vi "load_config.vi"(8 "error in (no error)":errorcluster, 11 "Path":path) -> (0 "error out":errorcluster, 3 "Config Settings":T1)   [LabVIEW 2024]
uses:
  controls/Config_Settings.ctl
  <vilib>/Utility/config.llb/Read Key (Double).vi
  <vilib>/Utility/config.llb/Read Key (U32).vi
  <vilib>/Utility/config.llb/NI_LVConfig.lvlib
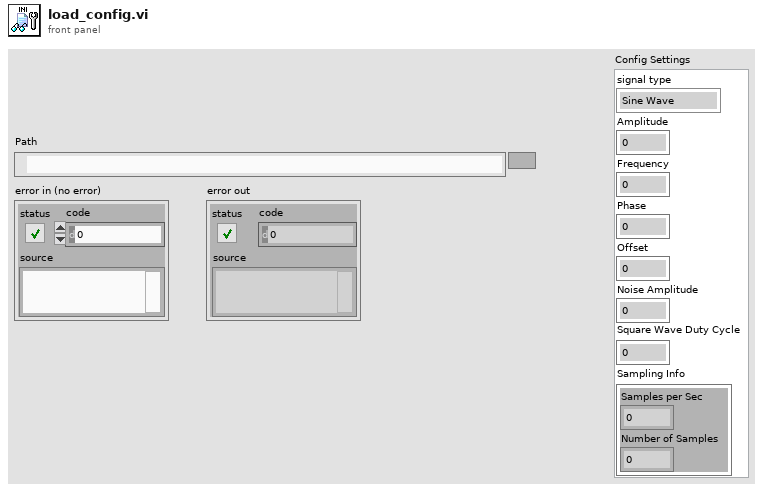
[diagram p1: front panel]
types:
  T1 = typedef "Config_Settings.ctl" = cluster{"signal type":enum16{"Sine Wave", "Triangle Wave", "Square Wave", "Sawtooth Wave"}, "Amplitude":dbl, "Frequency":dbl, "Phase":dbl, "Offset":dbl, "Noise Amplitude":dbl, "Square Wave Duty Cycle":dbl, "Sampling Info":cluster{"Samples per Sec":dbl, "Number of Samples":dbl}}
  T2 = enum16{"Sine Wave", "Triangle Wave", "Square Wave", "Sawtooth Wave"}
  T3 = typedef "NI_LVConfig.lvlib/Config Data RefNum.ctl" = refnum<k1>
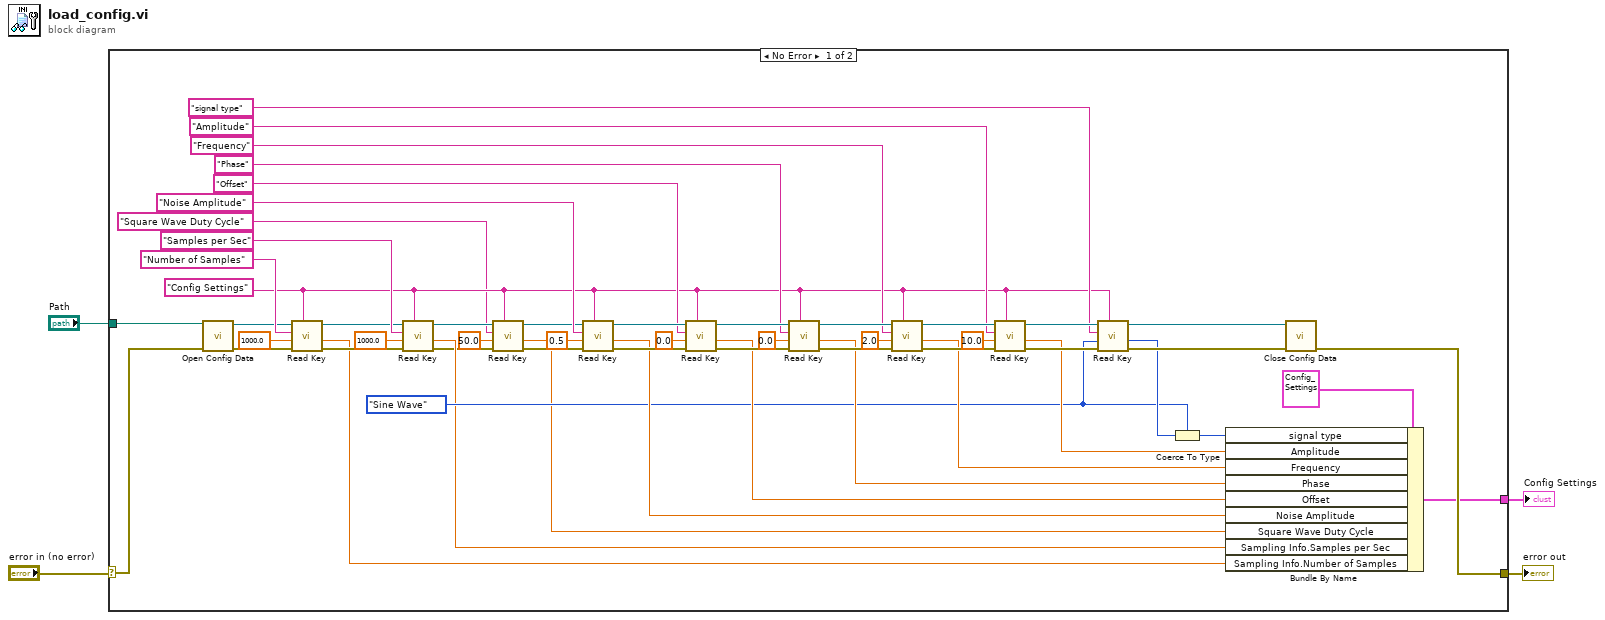
[diagram p0: block diagram]
diagram:
  n1 = case shown="No Error" "error in (no error)" {
    selector: "error in (no error)" -> [w46 w59]
    tunnel: [w45 w59] -> w4
    tunnel: [w43 _] -> w3
    tunnel: "Path" -> [w36 _]
    frame No Error {
      w28 = T2."Sine Wave" ("signal type")
      w7 = "Config Settings" ("section")
      n2 = call <vilib>:"Open Config Data.vi"("error in (no error)"=w46, "configuration file path"=w36) -> ("error out"=w21:errorcluster, "refnum"=w15:T3)  [unwired: 7 in, 1 out]
      n3 = call-poly <vilib>:"Read Key.vi"("section"=w7, "error in (no error)"=w21, "default value"=1000.0, "key"="Number of Samples", "refnum"=w15) -> ("error out"=w22:errorcluster, "value"=w13:dbl, "refnum out"=w16:T3)  [unwired: 3 in, 1 out]
      n4 = call-poly <vilib>:"Read Key.vi"("section"=w7, "error in (no error)"=w22, "default value"=1000.0, "key"="Samples per Sec", "refnum"=w16) -> ("error out"=w11:errorcluster, "value"=w14:dbl, "refnum out"=w12:T3)  [unwired: 3 in, 1 out]
      n5 = call-poly <vilib>:"Read Key.vi"("section"=w7, "error in (no error)"=w11, "default value"=50.0, "key"="Square Wave Duty Cycle", "refnum"=w12) -> ("error out"=w10:errorcluster, "value"=w5:dbl, "refnum out"=w9:T3)  [unwired: 3 in, 1 out]
      n6 = call-poly <vilib>:"Read Key.vi"("section"=w7, "error in (no error)"=w10, "default value"=0.5, "key"="Noise Amplitude", "refnum"=w9) -> ("error out"=w52:errorcluster, "value"=w30:dbl, "refnum out"=w58:T3)  [unwired: 3 in, 1 out]
      n7 = call-poly <vilib>:"Read Key.vi"("section"=w7, "error in (no error)"=w52, "default value"=0.0, "key"="Offset", "refnum"=w58) -> ("error out"=w51:errorcluster, "value"=w31:dbl, "refnum out"=w57:T3)  [unwired: 3 in, 1 out]
      n8 = call-poly <vilib>:"Read Key.vi"("section"=w7, "error in (no error)"=w51, "default value"=0.0, "key"="Phase", "refnum"=w57) -> ("error out"=w50:errorcluster, "value"=w32:dbl, "refnum out"=w56:T3)  [unwired: 3 in, 1 out]
      n9 = call-poly <vilib>:"Read Key.vi"("section"=w7, "error in (no error)"=w50, "default value"=2.0, "key"="Frequency", "refnum"=w56) -> ("error out"=w49:errorcluster, "value"=w33:dbl, "refnum out"=w55:T3)  [unwired: 3 in, 1 out]
      n10 = call-poly <vilib>:"Read Key.vi"("section"=w7, "error in (no error)"=w49, "default value"=10.0, "key"="Amplitude", "refnum"=w55) -> ("error out"=w48:errorcluster, "value"=w34:dbl, "refnum out"=w54:T3)  [unwired: 3 in, 1 out]
      n11 = call-poly <vilib>:"Read Key.vi"("section"=w7, "error in (no error)"=w48, "default value"=w28, "key"="signal type", "refnum"=w54) -> ("error out"=w47:errorcluster, "value"=w35:u32, "refnum out"=w53:T3)  [unwired: 3 in, 1 out]
      n12 = Coerce To Type(0:w35, 1:w28) -> (2:w29:T2)
      n13 = Bundle By Name(cluster=T1 {"signal type"=enum."Sine Wave", "Amplitude"=0.0, "Frequency"=0.0, "Phase"=0.0, "Offset"=0.0, "Noise Amplitude"=0.0, "Square Wave Duty Cycle"=0.0, "Sampling Info"={"Samples per Sec"=0.0, "Number of Samples"=0.0}} ("Config Settings"), "signal type"=w29, "Amplitude"=w34, "Frequency"=w33, "Phase"=w32, "Offset"=w31, "Noise Amplitude"=w30, "Square Wave Duty Cycle"=w5, "Sampling Info.Samples per Sec"=w14, "Sampling Info.Number of Samples"=w13) -> (w43:T1)
      n14 = call <vilib>:"Close Config Data.vi"("error in (no error)"=w47, "refnum"=w53) -> ("error out"=w45:errorcluster)  [unwired: 8 in, 1 out]
    }
    frame Error {
    }
  }
  "error out" <- w4
  "Config Settings" <- w3
